vi "choose_action.vi"(8 "Q":dbl[][](array[numeric]), 9 "state":dbl, 11 "epson":dbl) -> (2 "action":u8)   [LabVIEW 2022 SP3]
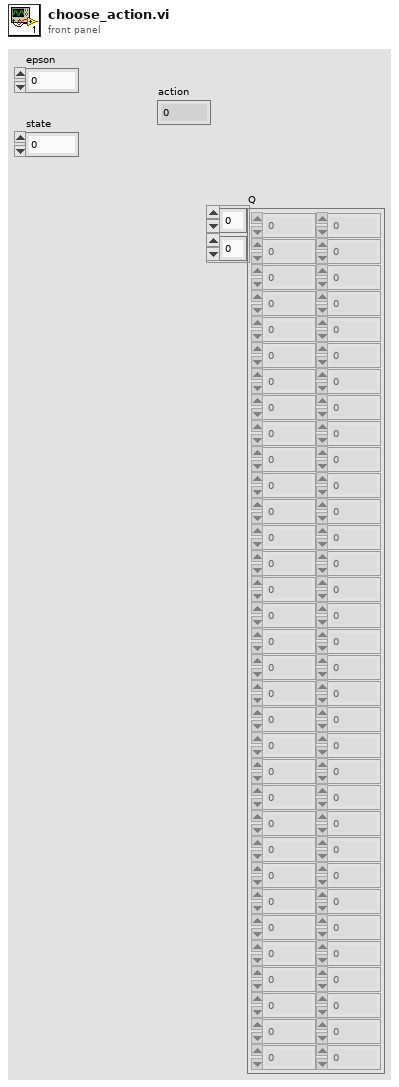
[diagram p1: front panel]
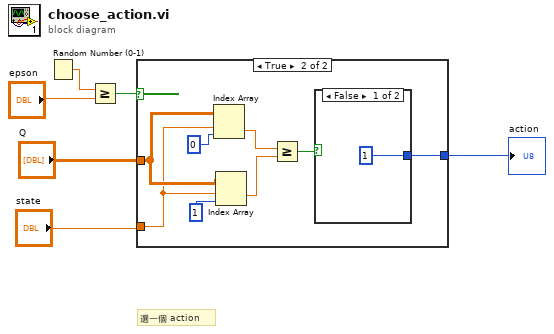
[diagram p0: block diagram]
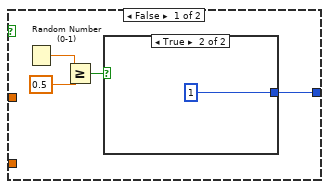
[diagram p2: hidden frame]
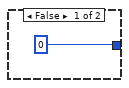
[diagram p3: hidden frame]
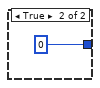
[diagram p4: hidden frame]
diagram:
  # "選一個 action"
  n1 = Random Number (0-1)() -> (number: 0 to 1=w2:dbl)
  n2 = Greater Or Equal?(x=w2, y="epson") -> (x >= y?=w6:bool)
  n3 = case shown="True" w6 {
    tunnel: "state" -> [_ w18]
    tunnel: "Q" -> [_ w19]
    tunnel: [w7 w13] -> w4
    frame False {
      n4 = Random Number (0-1)() -> (number: 0 to 1=w10:dbl)
      n5 = Greater Or Equal?(x=w10, y=0.5) -> (x >= y?=w8:bool)
      n6 = case shown="True" w8 {
        tunnel: [0 1] -> w7
        frame False {
        }
        frame True {
        }
      }
    }
    frame True {
      n7 = Index Array(array=w19, index (row)=w18, index (col)=0) -> (element=w16:dbl)
      n8 = Index Array(array=w19, index (row)=w18, index (col)=1) -> (element=w15:dbl)
      n9 = Greater Or Equal?(x=w16, y=w15) -> (x >= y?=w14:bool)
      n10 = case shown="False" w14 {
        tunnel: [1 0] -> w13
        frame False {
        }
        frame True {
        }
      }
    }
  }
  "action" <- w4
